vi "ConvertHexStrToHexData.vi"(11 "string":string) -> (3 "hex data":string)   [LabVIEW 2018, in "Library-DataConvert.lvlib"]
uses:
  Library-DataConvert.lvlib
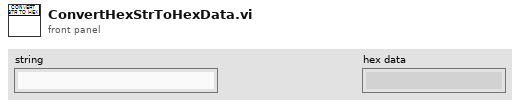
[diagram p1: front panel]
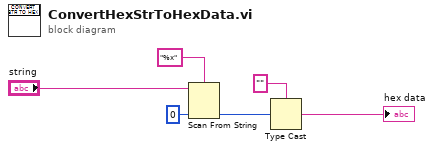
[diagram p0: block diagram]
diagram:
  n1 = Scan From String(format string="%x" ("포맷 문자열"), input string="string", default 1=u32 0 ("기본값 1")) -> (output 1=w4:u32)  [unwired: 2 in, 3 out]
  n2 = Type Cast(type="" ("타입"), x=w4) -> (*(type *) &x=→"hex data":string)
